vi "CalculateLabelPosition__slk_mt.vi"(6 "control? (t)":bool=TRUE, 7 "set label position configure":T1={"Control Label Position"="Left Middle", "Indicator Label Position"="Right Middle", "Apply to All"=FALSE}, 9 "label bounds":cluster{"Width":u32, "Height":u32}, 11 "master bounds rectangle":T2) -> (3 "label position":cluster{"Left":i32, "Top":i32})   [LabVIEW 2015, in "Lazyboots Menu Tool.lvlib"]
doc: "Gets label position with specified configurations."
uses:
  <vilib>/SLK/Lazyboots Menu Tool/Library/Lazyboots Menu Tool.lvlib
  <vilib>/SLK/Lazyboots Menu Tool/Private/SetLabelPosition/TypeDef/TypeDef_SetLabelPositionConfigure__slk_mt.ctl
panel:
  # "CalculateLabelPosition__slk_mt.vi\nGets label position with specified configurations.\n\nNOTICE -- YOU MUST LEAVE THIS NOTICE IN PLACE.\n\nCopyright (c) 2011, LIANG LIU Shawn.Liu.cn@gmail.com\nAll rights reserved.\n\nRedistribution and use in source and binary forms, with or without modification, are permitted provided that the following conditions are met:\n-Redistributions of source code must retain the above copyright notice, this list of conditions and the following disclaimer.\n-Redistributions in binary form must reproduce the above copyright notice, this list of conditions and the following disclaimer in the documentation and/or other materials provided with the distribution.\n-Neither the name of the eLp nor the names of its contributors may be used to endorse or promote products derived from this software without specific prior written permission.\n\nTHIS SOFTWARE IS PROVIDED BY THE COPYRIGHT HOLDERS AND CONTRIBUTORS \"AS IS\" AND ANY EXPRESS OR IMPLIED WARRANTIES, INCLUDING, BUT NOT LIMITED TO, THE IMPLIED WARRANTIES OF MERCHANTABILITY AND FITNESS FOR A PARTICULAR PURPOSE ARE DISCLAIMED. IN NO EVENT SHALL THE COPYRIGHT HOLDER OR CONTRIBUTORS BE LIABLE FOR ANY DIRECT, INDIRECT, INCIDENTAL, SPECIAL, EXEMPLARY, OR CONSEQUENTIAL DAMAGES (INCLUDING, BUT NOT LIMITED TO, PROCUREMENT OF SUBSTITUTE GOODS OR SERVICES; LOSS OF USE, DATA, OR PROFITS; OR BUSINESS INTERRUPTION) HOWEVER CAUSED AND ON ANY THEORY OF LIABILITY, WHETHER IN CONTRACT, STRICT LIABILITY, OR TORT (INCLUDING NEGLIGENCE OR OTHERWISE) ARISING IN ANY WAY OUT OF THE USE OF THIS SOFTWARE, EVEN IF ADVISED OF THE POSSIBILITY OF SUCH DAMAGE."
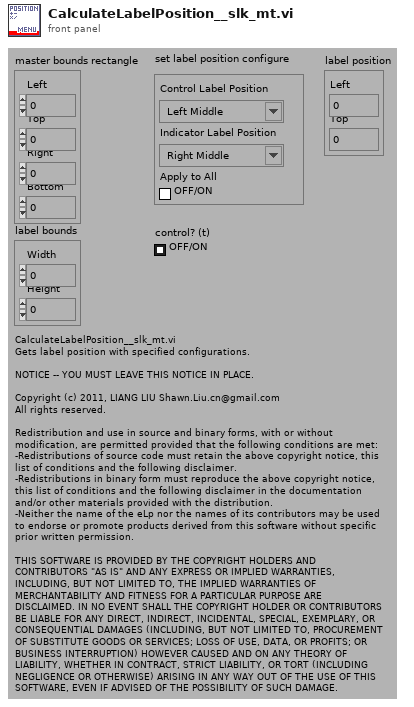
[diagram p1: front panel]
types:
  T1 = typedef "Lazyboots Menu Tool.lvlib/TypeDef_SetLabelPositionConfigure__slk_mt.ctl" = cluster{"Control Label Position":string, "Indicator Label Position":string, "Apply to All":bool}
  T2 = cluster{"Left":i16, "Top":i16, "Right":i16, "Bottom":i16}
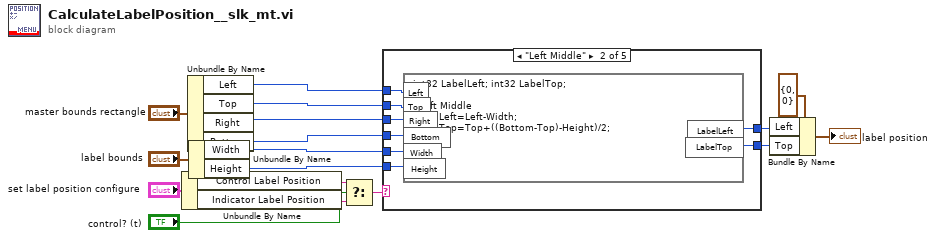
[diagram p0: block diagram]
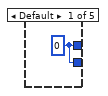
[diagram p2: hidden frame]
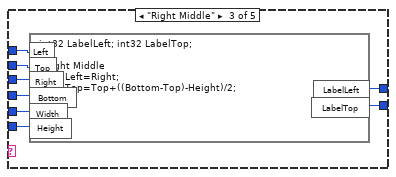
[diagram p3: hidden frame]
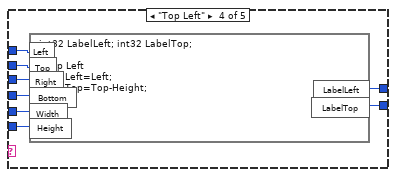
[diagram p4: hidden frame]
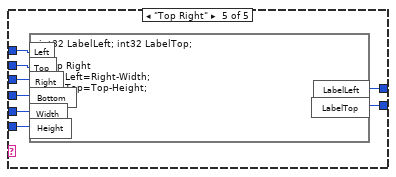
[diagram p5: hidden frame]
diagram:
  n1 = Unbundle By Name("set label position configure") -> ("Control Label Position"=w6:string, "Indicator Label Position"=w5:string)
  n2 = Unbundle By Name("master bounds rectangle") -> ("Left"=w17:i16, "Top"=w16:i16, "Right"=w15:i16, "Bottom"=w14:i16)
  n3 = Unbundle By Name("label bounds") -> ("Width"=w13:u32, "Height"=w12:u32)
  n4 = Select(t=w6, s="control? (t)", f=w5) -> (s? t:f=w4:string)
  n5 = case shown="\"Left Middle\"" w4 {
    tunnel: w17 -> [_ w26 w34 w42 w50]
    tunnel: w16 -> [_ w25 w33 w41 w49]
    tunnel: w15 -> [_ w24 w32 w40 w48]
    tunnel: w14 -> [_ w23 w31 w39 w47]
    tunnel: w13 -> [_ w22 w30 w38 w46]
    tunnel: w12 -> [_ w21 w29 w37 w45]
    tunnel: [w18 w20 w28 w36 w44] -> w9
    tunnel: [w18 w19 w27 w35 w43] -> w8
    frame Default {
      w18 = 0
    }
    frame "Left Middle" {
      n6 = formula code="int32 LabelLeft; int32 LabelTop;\n\n//Left Middle\nLabelLeft=Left-Width;\nLabelTop=Top+((Bottom-Top)-Height)/2;"("Left"=w26, "Top"=w25, "Right"=w24, "Bottom"=w23, "Width"=w22, "Height"=w21) -> ("LabelLeft"=w20:i32, "LabelTop"=w19:i32)
    }
    frame "Right Middle" {
      n7 = formula code="int32 LabelLeft; int32 LabelTop;\n\n//Right Middle\nLabelLeft=Right;\nLabelTop=Top+((Bottom-Top)-Height)/2;"("Left"=w34, "Top"=w33, "Right"=w32, "Bottom"=w31, "Width"=w30, "Height"=w29) -> ("LabelLeft"=w28:i32, "LabelTop"=w27:i32)
    }
    frame "Top Left" {
      n8 = formula code="int32 LabelLeft; int32 LabelTop;\n\n//Top Left\nLabelLeft=Left;\nLabelTop=Top-Height;"("Left"=w42, "Top"=w41, "Right"=w40, "Bottom"=w39, "Width"=w38, "Height"=w37) -> ("LabelLeft"=w36:i32, "LabelTop"=w35:i32)
    }
    frame "Top Right" {
      n9 = formula code="int32 LabelLeft; int32 LabelTop;\n\n//Top Right\nLabelLeft=Right-Width;\nLabelTop=Top-Height;"("Left"=w50, "Top"=w49, "Right"=w48, "Bottom"=w47, "Width"=w46, "Height"=w45) -> ("LabelLeft"=w44:i32, "LabelTop"=w43:i32)
    }
  }
  n10 = Bundle By Name(cluster=cluster{"Left":i32, "Top":i32} {"Left"=0, "Top"=0} ("Label.Position"), "Left"=w9, "Top"=w8) -> (→"label position":cluster{"Left":i32, "Top":i32})
